vi "Matrix_display_host.vi"() -> ()   [LabVIEW 2018]
uses:
  <vilib>/userdefined/High Color/nirio_resource_hc.ctl
  <vilib>/FPGAPlugInAG/PXI-7953R/niLvFpga_Open_PXI-7953R.vi
  <vilib>/rvi/interface/common/dynamic/niFpgaDynamicAddResources.vi
  <vilib>/FPGAPlugInAG/Dynamic/niLvFpga_Reset_Dynamic.vi
  <vilib>/FPGAPlugInAG/Dynamic/niLvFpga_Run_Dynamic.vi
  <vilib>/Utility/error.llb/Error Cluster From Error Code.vi
  <vilib>/rvi/errors/niLvFpgaAdjustHostInterfaceError.vi
  <vilib>/FPGAPlugInAG/Dynamic/niLvFpga_Close_Dynamic.vi
  <vilib>/rvi/interface/nirviOpenFPGA/nirviOpenFPGA.xnode
  FPGA Bitfiles/Matrix_Writetarget_Matrixdisplaytar_dItzC8vODKI.lvbitx
  <vilib>/rvi/interface/nirviMethod/nirviMethod.xnode
  <vilib>/rvi/interface/nirviReadWriteControl/nirviReadWriteControl.xnode
  <vilib>/rvi/interface/nirviCloseFPGA/nirviCloseFPGA.xnode
  <vilib>/FPGAPlugInAG/Dynamic/niLvFpga_ReadFifo_Dynamic.vi
  <vilib>/rvi/errors/niLvFpgaMergeErrorWithErrorCode.vi
  NiFpgaLv.dll
  <vilib>/rvi/interface/Simulation/niFpgaSimulationCallBeginRW.vi
panel:
  out "Max":u32
  in  "y":bool=TRUE
  out "Elements Remaining 2":u32
  in  "2574_2xNumPix":i32
  in  "1_Pix_counter":i16
  out "Elements Remaining":u32
  out "Data":i16[](array[numeric])
  in  "ReadDRAM":bool
  in  "AddressRead":u32
  out "DataOut":i16
  in  "DataIn":i16
  in  "AddressWrite":u32
  in  "stop":bool
  in  "Number of Elements":u32
  in  "1_EXTCLK_divider":i16
  in  "resource name":T1 caption="RIO Device"
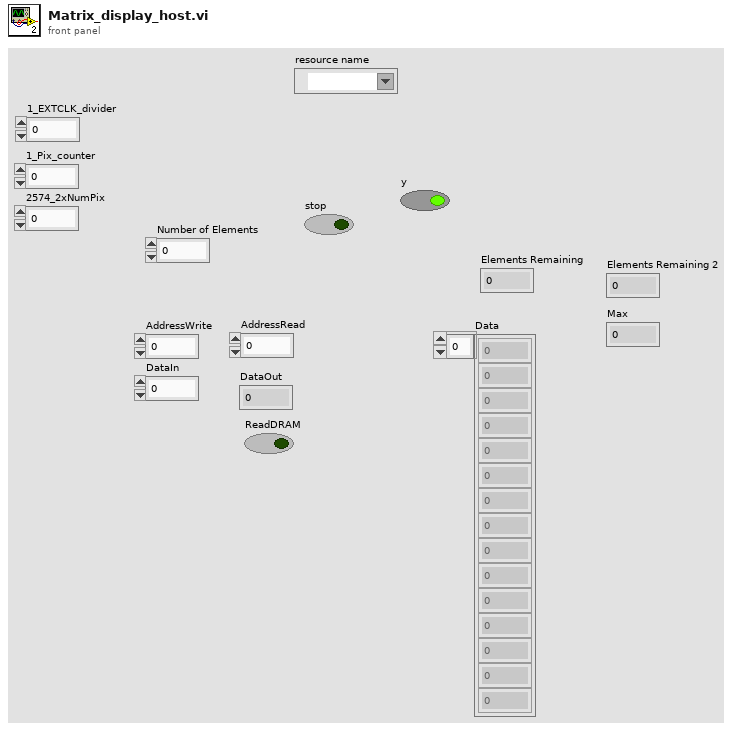
[diagram p1: front panel]
types:
  T1 = typedef "nirio_resource_hc.ctl" = tag
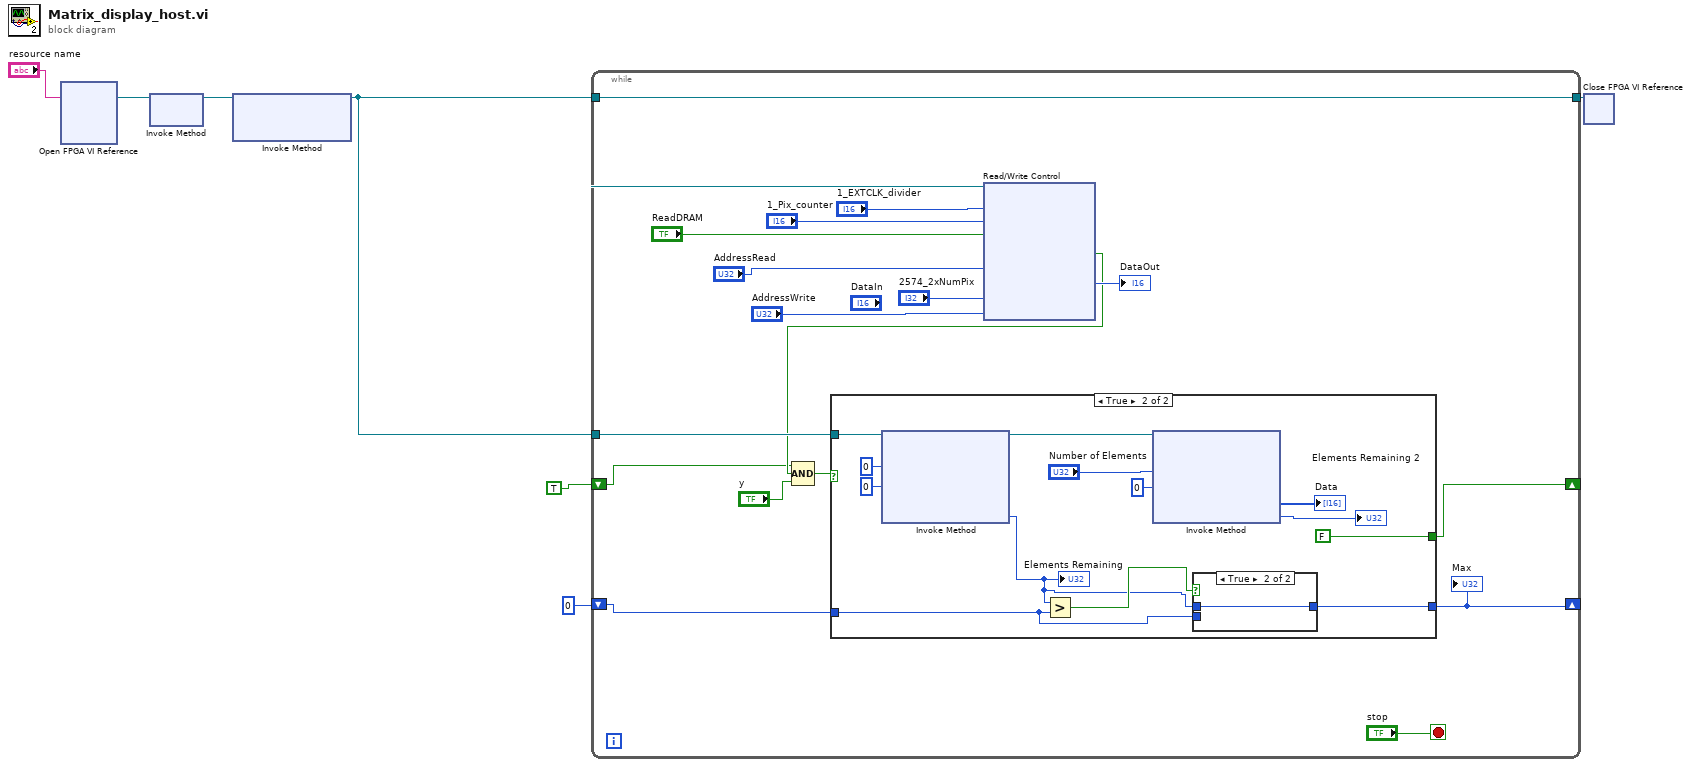
[diagram p0: block diagram]
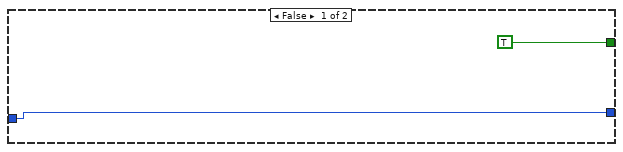
[diagram p2: hidden frame]
diagram:
  n1 = xnode "Open FPGA VI Reference"("resource name"="resource name") -> ("FPGA VI Reference Out"=w7:refnum<k20>)  [unwired: 1 in, 1 out]
  n2 = xnode "Invoke Method"("FPGA VI Reference In"=w7) -> ("FPGA VI Reference Out"=w6:refnum<k20>)  [unwired: 1 in, 1 out]
  n3 = xnode "Invoke Method"("FPGA VI Reference In"=w6) -> ("FPGA VI Reference Out"=w3:refnum<k20>)  [unwired: 2 in, 1 out]
  n4 = while {
    tunnel: w3 -> [w23]
    tunnel: [w23] -> w5
    tunnel: w3 -> [w22]
    shift-right: [w15] -> _
    shift-left: TRUE -> [w10]
    shift-right: [w8] -> _
    shift-left: 0 -> [w9]
    stop <- "stop" stop-if-true
    n5 = xnode "Read/Write Control"("FPGA VI Reference In"=w23, "1_EXTCLK_divider"="1_EXTCLK_divider", "1_Pix_counter"="1_Pix_counter", "Read"="ReadDRAM", "AddressRead"="AddressRead", "2574_2xNumPix"="2574_2xNumPix", "AddressWrite"="AddressWrite") -> ("line_ready"=w12:bool, "DataOut"=→"DataOut":i16)  [unwired: 1 in, 2 out]
    n6 = Compound Arithmetic op=AND(w10, w12, "y") -> (w16:bool)
    n7 = case shown="True" w16 {
      tunnel: w22 -> [_ w39]
      tunnel: [TRUE FALSE] -> w15
      tunnel: w9 -> [w25 w27]
      tunnel: [w25 w28] -> w8
      frame False {
      }
      frame True {
        n8 = xnode "Invoke Method"("FPGA VI Reference In"=w39, "Number of Elements"=u32 0, "Timeout (ms)"=0) -> ("FPGA VI Reference Out"=w38:refnum<k20>, "Elements Remaining"=w29:u32)  [unwired: 1 in, 2 out]
        "Elements Remaining" <- w29
        n9 = Greater?(x=w29, y=w27) -> (0:w30:bool)
        n10 = xnode "Invoke Method"("FPGA VI Reference In"=w38, "Number of Elements"="Number of Elements", "Timeout (ms)"=0) -> ("Data"=→"Data":u16[], "Elements Remaining"=→"Elements Remaining 2":u32)  [unwired: 1 in, 2 out]
        n11 = case shown="True" w30 {
          tunnel: w29 -> [_ w41]
          tunnel: [w40 w41] -> w28
          tunnel: w27 -> [w40 _]
          frame False {
          }
          frame True {
          }
        }
      }
    }
    "Max" <- w8
  }
  n12 = xnode "Close FPGA VI Reference"("FPGA VI Reference In"=w5) -> ()  [unwired: 1 in, 1 out]
